vi "tdmsGenToolAllDAQmxTypes.vi"() -> ()   [LabVIEW 2026]
uses:
  <vilib>/Platform/TimedLoop/XDataNode/nitl_modes.ctl
  <vilib>/Platform/TimedLoop/XDataNode/timing_clust.ctl
  <vilib>/Platform/TimedLoop/XDataNode/wakeup.ctl
  <vilib>/DAQmx/read.llb/DAQmx Read (Analog 1D DBL 1Chan NSamp).vi
  <vilib>/DAQmx/create/channels.llb/DAQmx Create Channel (AI-Current-Basic).vi
  <vilib>/DAQmx/create/channels.llb/DAQmx Create Channel (AI-Temperature-RTD).vi
  <vilib>/DAQmx/create/channels.llb/DAQmx Create Channel (AI-Temperature-Thermocouple).vi
  <vilib>/DAQmx/create/channels.llb/DAQmx Create Channel (AI-Strain-Strain Gage).vi
  <vilib>/DAQmx/configure/timing.llb/DAQmx Timing (Sample Clock).vi
  <vilib>/DAQmx/configure/task.llb/DAQmx Configure Logging (TDMS).vi
  <vilib>/DAQmx/miscellaneous.llb/DAQmx Fill In Error Info.vi
  <vilib>/platform/TimedLoop/XDataNode/XDataNode.xnode
  <vilib>/DAQmx/create/channels.llb/DAQmx Create Channel (AI-Voltage-Basic).vi
  <vilib>/DAQmx/create/scale.llb/DAQmx Create Scale (Linear).vi
  <vilib>/Platform/TimedLoop/XDataNode/XDNodeRunTimeDep.lvlib
  <resource>/objmgr/daqmx.rc
panel:
  in  "DAQType Enum":T1(ring)
  in  "double?":bool
  in  "file format version (2.0)":enum16{"1.0", "2.0"}(ring)=enum."2.0"
  in  "create index file? (T)":bool=TRUE
  in  "byte order (2:little-endian)":T2(ring)
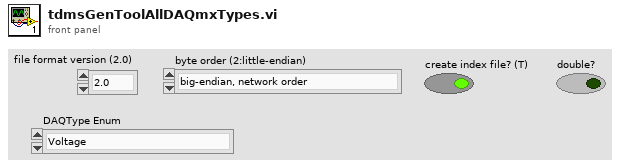
[diagram p1: front panel]
types:
  T1 = enum16{"Voltage", "Current", "RTD", "Thermocouple", "Strain"}
  T2 = enum16{"big-endian, network order", "native, host order", "little-endian"}
  T3 = typedef "XDNodeRunTimeDep.lvlib/nitl_modes.ctl" = enum32{"No Change", "Process missed periods, maintain original phase", "Discard missed periods, maintain original phase", "Process missed periods, ignore original phase", "Discard missed periods, ignore original phase"}
  T4 = cluster{"gage factor":dbl, "nominal gage resistance":dbl, "poisson ratio":dbl}
  T5 = typedef "XDNodeRunTimeDep.lvlib/timing_clust.ctl" = cluster{"Expected End [f-1]":u64, "Actual End [f-1]":u64, "Finished Late? [f-1]":bool, "Expected End [i-1]":u64, "Actual End [i-1]":u64, "Finished Late? [i-1]":bool, "Expected Start [i]":u64, "Actual Start [i]":u64, "Expected Start [f]":u64, "Actual Start [f]":u64, "Source Name":string, "Structure Name":string, "Period":i64, "Deadline":i64, "Offset":i64, "Start":i64, "Priority":i32, "Timeout":i32, "Mode":T3, "Wakeup Reason":T6, "Error":errorcluster, "Source Type":string, "Secondary Source Type":string, "Global End Time":u64, "Global Start Time":u64, "Frame Duration":u64, "Iteration Duration":u64, "Assigned CPU":i32, "I/O Scan Engine Mode":u32}
  T6 = typedef "XDNodeRunTimeDep.lvlib/wakeup.ctl" = enum32{"Normal", "Aborted", "Asynchronous wakeup", "Timing source error", "Timed loop error", "Timeout"}
  T7 = enum16{"open", "open or create", "create or replace", "create", "open (read-only)"}
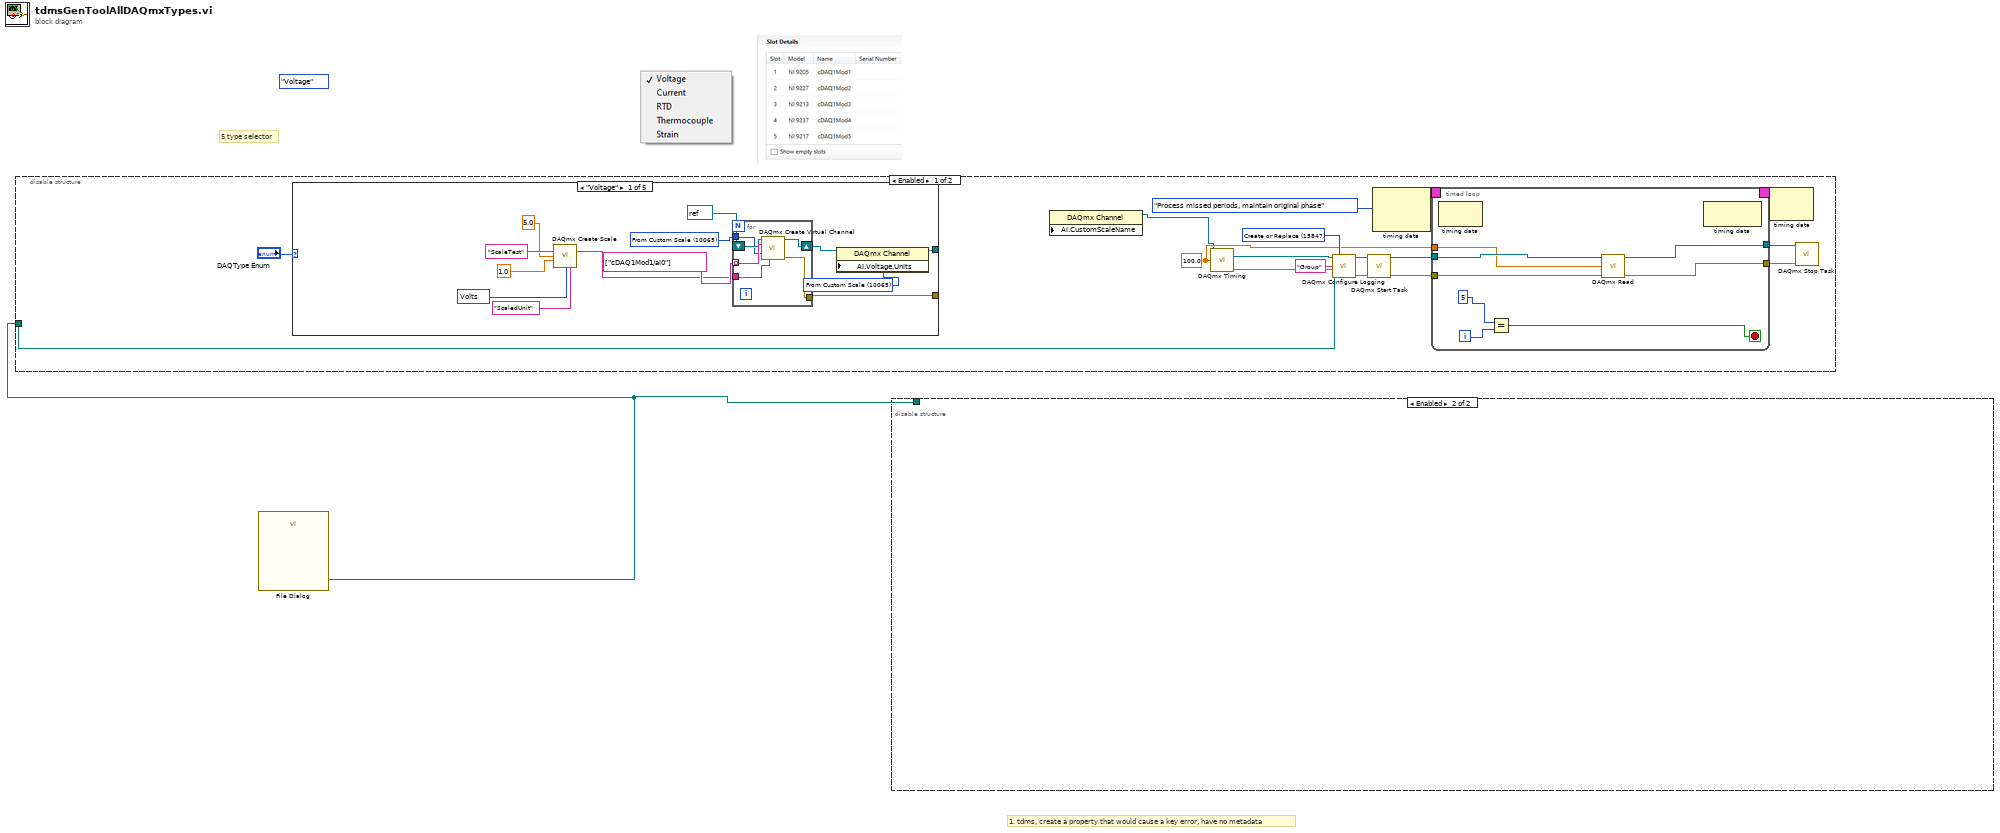
[diagram p0: block diagram]
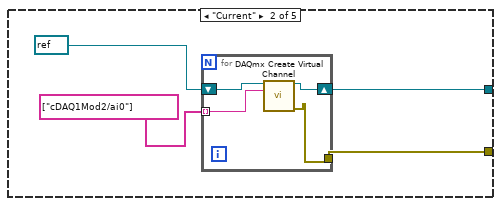
[diagram p2: hidden frame]
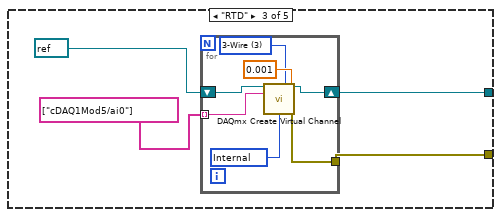
[diagram p3: hidden frame]
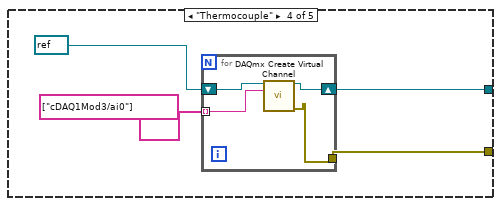
[diagram p4: hidden frame]
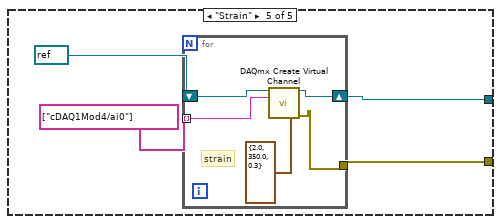
[diagram p5: hidden frame]
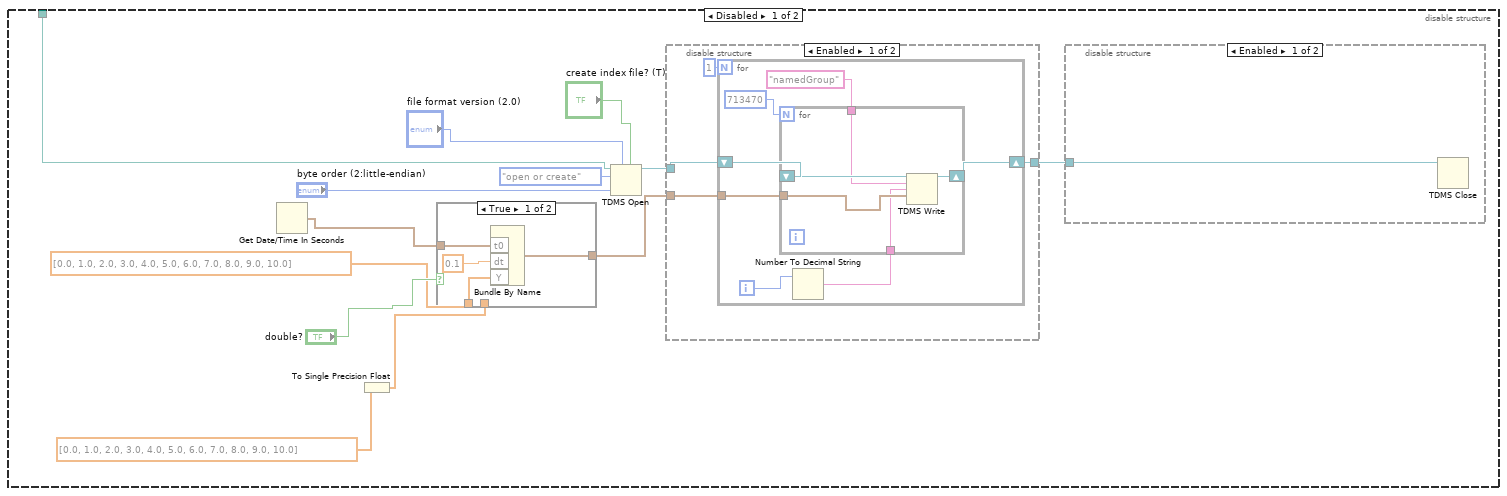
[diagram p7: hidden frame]
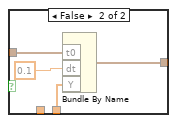
[diagram p10: hidden frame]
diagram:
  (unwired) T1."Voltage"
  # "5 type selector"
  # "1. tdms, create a property that would cause a key error, have no metadata"
  n1 = call "File Dialog"() -> ("selected path"=w1:path)  [unwired: 12 in, 3 out]
  n2 = disable-structure shown="Enabled" {
    disable-tunnel: w1 -> [w4 _]
    frame Enabled {
      w16 = 15847 items=["Open"=10437, "Open or Create"=15846, "Create or Replace"=15847, "Create"=15848] ("operation")
      w3 = 100.0 ("rate")
      n3 = case shown="\"Voltage\"" "DAQType Enum" {
        tunnel: [w26 w41 w49 w60 w65] -> _
        tunnel: [w31 w40 w48 w59 w68] -> _
        frame "Voltage" {
          w25 = 10065 items=["Volts"=10348, "From Custom Scale"=10065, "From TEDS"=12516] ("AI.Voltage.Units")
          w19 = 10348 items=["Volts"=10348, "Amps"=10342, "Watts"=16203, "Deg F"=10144, "Deg C"=10143, "Deg R"=10145, "Kelvins"=10325, "Strain"=10299, "Ohms"=10384, "Hz"=10373, "Seconds"=10364, "Meters"=10219, "Inches"=10379, "Degrees"=10146, "Radians"=10273, "Ticks"=10304, "g"=10186, "m/s^2"=12470, "m/s"=15959, "in/s"=15960, "Pascals"=10081, "Newtons"=15875, "Pounds"=15876, "kgf"=15877, "psi"=15879, "bar"=15880, "Nm"=15881, "oz-in"=15882, "lb-in"=15883, "lb-ft"=15884, "Volts/Volt"=15896, "mVolts/Volt"=15897, "pCoulombs"=16103, "Coulombs"=16102, "From TEDS"=12516] ("pre-scaled units")
          w28 = 10065 items=["Volts"=10348, "From Custom Scale"=10065] ("units")
          n4 = call-poly <vilib>:"DAQmx Create Scale.vi"("name"="ScaleTest", "slope"=5.0, "y-intercept"=1.0, "pre-scaled units"=w19, "scaled units"="ScaledUnit") -> ("scale out"=w20:tag)  [unwired: 9 in, 1 out]
          n5 = for {
            tunnel: [w36] -> w31
            tunnel: tag[] ["cDAQ1Mod1/ai0"] ("Voltage Channels") -> [w35] mode=indexing
            shift-right: [w37] -> w27
            shift-left: refnum<k21> refnum ("task out") -> [w34]
            tunnel: w28 -> [w33]
            tunnel: w20 -> [w32]
            n6 = call-poly <vilib>:"DAQmx Create Virtual Channel.vi"("task in"=w34, "physical channels"=w35, "units"=w33, "custom scale name"=w32) -> ("task out"=w37:refnum<k21>, "error out"=w36:errorcluster)  [unwired: 10 in]
          }
          n7 = property class="DAQmx Channel"(reference=w27, "AI.Voltage.Units"=w25) -> (reference out=w26:refnum<k21>)  [unwired: 1 in, 1 out]
        }
        frame "Current" {
          n8 = for {
            tunnel: [w44] -> w40
            tunnel: tag[] ["cDAQ1Mod2/ai0"] ("Voltage Channels") -> [w43] mode=indexing
            shift-right: [w45] -> w41
            shift-left: refnum<k21> refnum ("task out") -> [w42]
            n9 = call-poly <vilib>:"DAQmx Create Virtual Channel.vi"("task in"=w42, "physical channels"=w43) -> ("task out"=w45:refnum<k21>, "error out"=w44:errorcluster)  [unwired: 12 in]
          }
        }
        frame "RTD" {
          n10 = for {
            tunnel: [w55] -> w48
            tunnel: tag[] ["cDAQ1Mod5/ai0"] ("Voltage Channels") -> [w54] mode=indexing
            shift-right: [w56] -> w49
            shift-left: refnum<k21> refnum ("task out") -> [w53]
            w50 = 3 items=["2-Wire"=2, "3-Wire"=3, "4-Wire"=4] ("resistance configuration")
            w52 = 10200 items=["Internal"=10200, "External"=10167, "None"=10230] ("current excitation source")
            n11 = call-poly <vilib>:"DAQmx Create Virtual Channel.vi"("task in"=w53, "resistance configuration"=w50, "physical channels"=w54, "current excitation value"=0.001, "current excitation source"=w52) -> ("task out"=w56:refnum<k21>, "error out"=w55:errorcluster)  [unwired: 9 in]
          }
        }
        frame "Thermocouple" {
          n12 = for {
            tunnel: [w63] -> w59
            tunnel: tag[] ["cDAQ1Mod3/ai0"] ("Voltage Channels") -> [w62] mode=indexing
            shift-right: [w64] -> w60
            shift-left: refnum<k21> refnum ("task out") -> [w61]
            n13 = call-poly <vilib>:"DAQmx Create Virtual Channel.vi"("task in"=w61, "physical channels"=w62) -> ("task out"=w64:refnum<k21>, "error out"=w63:errorcluster)  [unwired: 12 in]
          }
        }
        frame "Strain" {
          n14 = for {
            tunnel: [w72] -> w68
            tunnel: tag[] ["cDAQ1Mod4/ai0"] ("Voltage Channels") -> [w71] mode=indexing
            shift-right: [w73] -> w65
            shift-left: refnum<k21> refnum ("task out") -> [w70]
            # "strain"
            n15 = call-poly <vilib>:"DAQmx Create Virtual Channel.vi"("task in"=w70, "physical channels"=w71, "strain gage information"=T4 {"gage factor"=2.0, "nominal gage resistance"=350.0, "poisson ratio"=0.3}) -> ("task out"=w73:refnum<k21>, "error out"=w72:errorcluster)  [unwired: 11 in]
          }
        }
      }
      n16 = property class="DAQmx Channel" props=["AI.CustomScaleName"]() -> (reference out=w2:refnum<k21>)  [unwired: 3 in, 1 out]
      n17 = call-poly <vilib>:"DAQmx Timing.vi"("task/channels in"=w2, "rate"=w3) -> ("task out"=w14:refnum<k21>, "error out"=w13:errorcluster)  [unwired: 12 in]
      n18 = call-poly <vilib>:"DAQmx Configure Logging.vi"("task/channels in"=w14, "operation"=w16, "file path"=w4, "group name"="Group", "error in"=w13) -> ("task out"=w12:refnum<k21>, "error out"=w11:errorcluster)  [unwired: 9 in]
      n19 = call <vilib>:"DAQmx Start Task.vi"("task/channels in"=w12, "error in"=w11) -> ("task out"=w10:refnum<k21>, "error out"=w9:errorcluster)  [unwired: 12 in]
      n20 = node-c288(nitl_modes."Process missed periods, maintain original phase" ("Mode")) -> (w18:T5)  [unwired: 1 in]
      n21 = timed-loop {
        tunnel: w10 -> [w78]
        tunnel: w9 -> [w77]
        timing: w18 -> [_]
        timing-out: [_] -> w17
        tunnel: [w76] -> w8
        tunnel: [w75] -> w7
        tunnel: w3 -> [w74]
        i -> [w81]
        stop <- w80 stop-if-true
        n22 = node-c288() -> ()  [unwired: 1 in, 1 out]
        n23 = Equal?(x=5, y=w81) -> (x = y?=w80:bool)
        n24 = call-poly <vilib>:"DAQmx Read.vi"("task/channels in"=w78, "number of samples per channel"=w74, "error in"=w77) -> ("task out"=w76:refnum<k21>, "error out"=w75:errorcluster)  [unwired: 10 in, 1 out]
        n25 = node-c288() -> ()  [unwired: 1 in, 1 out]
      }
      n26 = node-c288(w17) -> ()  [unwired: 1 out]
      n27 = call <vilib>:"DAQmx Stop Task.vi"("task/channels in"=w8, "error in"=w7) -> ()  [unwired: 12 in, 2 out]
    }
    frame Disabled {
    }
  }
  n28 = disable-structure shown="Enabled" {
    disable-tunnel: w1 -> [w98 _]
    frame Disabled {
      n29 = Get Date/Time In Seconds() -> (seconds since 1Jan1904=w91:timestamp)
      n30 = To Single Precision Float(number=dbl[] [0.0, 1.0, 2.0, 3.0, 4.0, 5.0, 6.0, 7.0, 8.0, 9.0, 10.0] ("Y")) -> (single precision float=w92:sgl[])
      n31 = case shown="True" "double?" {
        tunnel: w91 -> [w122 w126]
        tunnel: [w120 w124] -> w89
        tunnel: dbl[] [0.0, 1.0, 2.0, 3.0, 4.0, 5.0, 6.0, 7.0, 8.0, 9.0, 10.0] ("Y") -> [w119 _]
        tunnel: w92 -> [_ w123]
        frame True {
          n32 = Bundle By Name("t0"=w122, "dt"=0.1, "Y"=w119) -> (w120:waveform(dbl))  [unwired: 1 in]
        }
        frame False {
          n33 = Bundle By Name("t0"=w126, "dt"=0.1, "Y"=w123) -> (w124:waveform(sgl))  [unwired: 1 in]
        }
      }
      n34 = TDMS Open(5:"create index file? (T)", 7:"file format version (2.0)", 9:"byte order (2:little-endian)", 10:T7."open or create" ("operation (0:open)"), 11:w98) -> (3:w100:refnum<k34>)  [unwired: 2 in, 1 out]
      n35 = disable-structure shown="Enabled" {
        disable-tunnel: w100 -> [w104 w117]
        disable-tunnel: [w103 w117] -> w90
        disable-tunnel: w89 -> [w102 _]
        frame Enabled {
          n36 = for {
            N: 1 -> [_]
            tunnel: w102 -> [w107]
            shift-right: [w110] -> w103
            shift-left: w104 -> [w111]
            i -> [w106]
            n37 = Number To Decimal String(number=w106) -> (decimal integer string=w105:string)  [unwired: 1 in]
            n38 = for {
              N: 713470 -> [_]
              shift-right: [w115] -> w110
              shift-left: w111 -> [w116]
              tunnel: "namedGroup" ("group name in (Untitled)") -> [w114]
              tunnel: w107 -> [w113]
              tunnel: w105 -> [w112]
              n39 = TDMS Write(0:w116, 5:w114, 7:w112, 9:w113) -> (4:w115:refnum<k34>)  [unwired: 2 in, 3 out]
            }
          }
        }
        frame Disabled {
        }
      }
      n40 = disable-structure shown="Enabled" {
        disable-tunnel: w90 -> [w118 _]
        frame Enabled {
          n41 = TDMS Close(11:w118) -> ()  [unwired: 1 in, 2 out]
        }
        frame Disabled {
        }
      }
    }
    frame Enabled {
    }
  }
